vi "Get Remaing System Actions.vi"(8 "error in (no error)":errorcluster, 11 "TLB` Error Handler in":refnum<class "TLB` Error Handler.lvclass">) -> (0 "error out":errorcluster, 2 "Remaing System Actions":string[](array[string]), 3 "TLB` Error Handler out":refnum<class "TLB` Error Handler.lvclass">)   [LabVIEW 2015, in "TLB` Template.lvlib" / "TLB` Error Handler.lvclass"]
uses:
  TLB` Error Handler.lvclass
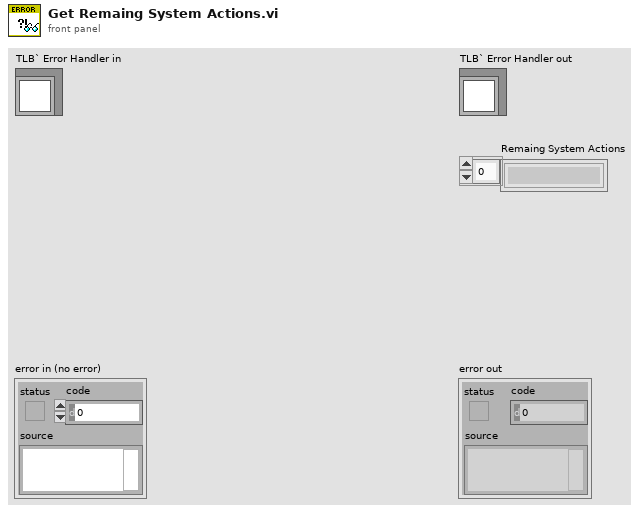
[diagram p1: front panel]
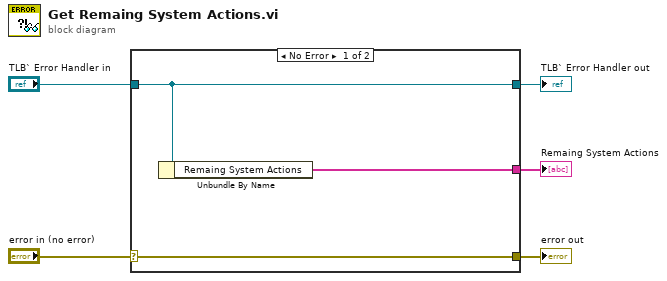
[diagram p0: block diagram]
diagram:
  n1 = case shown="No Error" "error in (no error)" {
    selector: "error in (no error)" -> [w8 w9]
    tunnel: [w8 w9] -> w4
    tunnel: [w7 w10] -> w2
    tunnel: "TLB` Error Handler in" -> [w7 w10]
    tunnel: [w6 _] -> w1
    frame No Error {
      n2 = Unbundle By Name(w7) -> ("Remaing System Actions"=w6:string[])
    }
    frame Error {
    }
  }
  "error out" <- w4
  "TLB` Error Handler out" <- w2
  "Remaing System Actions" <- w1
